vi "Realsense Cam Stream Restart All.vi"(8 "error in (no error)":errorcluster, 11 "Realsense Cam in":refnum<class "Realsense Cam.lvclass">) -> (0 "error out":errorcluster, 3 "Realsense Cam out":refnum<class "Realsense Cam.lvclass">)   [LabVIEW 2018, in "Realsense Cam.lvclass"]
uses:
  Realsense Cam.lvclass
  Realsense Cam.lvclass/Realsense Cam.ctl
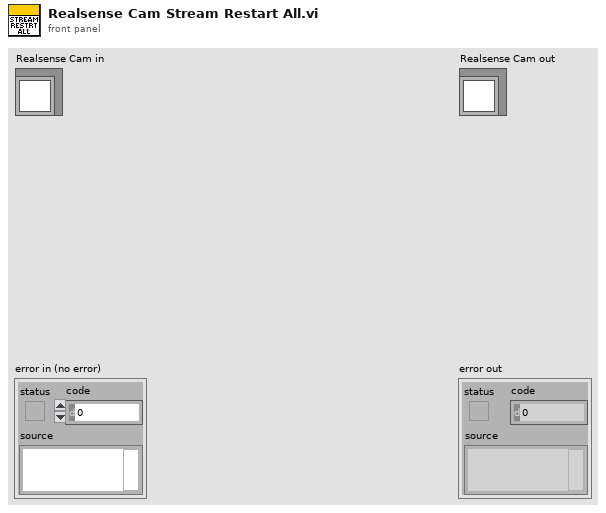
[diagram p1: front panel]
types:
  T1 = cluster{"Depth?":bool, "Left IR?":bool, "Left IR Unrectified?":bool, "Right IR?":bool, "Right IR Unrectified?":bool, "Color?":bool, "RGB Ext.?":bool}
  T2 = typedef "Realsense Cam.lvclass/Activated Stream STYP.ctl" = cluster{"Stream Config":T3, "Profile Handle":u64, "Stream":T5}
  T3 = typedef "Realsense Cam.lvclass/Stream Config STYP.ctl" = cluster{"Stream Type":T4, "Resolution":u16}
  T4 = typedef "Realsense Cam.lvclass/Stream Types Enum STYP.ctl" = enum16{"Depth", "Left IR", "Left IR Unrectified", "Right IR", "Right IR Unrectified", "Color", "RGB Ext."}
  T5 = typedef "Realsense Cam.lvclass/Stream STYP.ctl" = cluster{"Strings":string[], "Intrinsics":cluster{"width":i32, "height":i32, "fps":i32, "Profile":u64, "ppx":sgl, "ppy":sgl, "fx":sgl, "fy":sgl, "model":u32}[], "Current Data":T6}
  T6 = typedef "Realsense Cam.lvclass/Stream Frame Data STYP.ctl" = cluster{"Depths":sgl[][], "Bytes":u8[], "16-Bit IR":u16[], "Height":i32, "Width":i32}
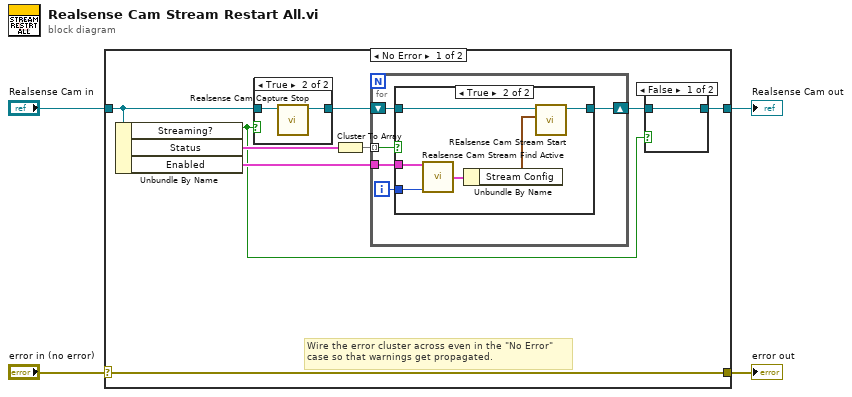
[diagram p0: block diagram]
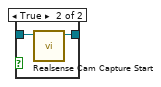
[diagram p2: hidden frame]
diagram:
  n1 = case shown="No Error" "error in (no error)" {
    selector: "error in (no error)" -> [w13 w33]
    tunnel: [w13 w33] -> w3
    tunnel: [w6 w32] -> w1
    tunnel: "Realsense Cam in" -> [w9 w32]
    frame No Error {
      # "Wire the error cluster across even in the \"No Error\"\ncase so that warnings get propagated."
      n2 = Unbundle By Name(w9) -> ("Streaming?"=w5:bool, "Status"=w12:T1, "Enabled"=w10:T2[])
      n3 = case shown="True" w5 {
        tunnel: w9 -> [w17 w19]
        tunnel: [w17 w18] -> w8
        frame False {
        }
        frame True {
          n4 = call-dynamic "Realsense Cam Capture Stop.vi"("Realsense Cam in"=w19) -> ("Realsense Cam out"=w18:refnum<class "Realsense Cam.lvclass">)  [unwired: 8 in, 2 out]
        }
      }
      n5 = Cluster To Array(cluster=w12) -> (array=w11:bool[])
      n6 = for {
        tunnel: w11 -> [w21] mode=indexing
        shift-right: [w20] -> w7
        shift-left: w8 -> [w24]
        tunnel: w10 -> [w23]
        i -> [w22]
        n7 = case shown="True" w21 {
          tunnel: w24 -> [w25 w31]
          tunnel: w23 -> [_ w30]
          tunnel: w22 -> [_ w27]
          tunnel: [w25 w28] -> w20
          frame False {
          }
          frame True {
            n8 = call "Realsense Cam Stream Find Active.vi"("Streams"=w30, "Stream Types"=w27) -> ("Activated Stream"=w29:T2)  [unwired: 11 in, 2 out]
            n9 = Unbundle By Name(w29) -> ("Stream Config"=w26:T3)
            n10 = call-dynamic "REalsense Cam Stream Start.vi"("Stream Config"=w26, "Realsense Cam in"=w31) -> ("Realsense Cam out"=w28:refnum<class "Realsense Cam.lvclass">)  [unwired: 8 in, 1 out]
          }
        }
      }
      n11 = case shown="False" w5 {
        tunnel: w7 -> [w14 w16]
        tunnel: [w14 w15] -> w6
        frame False {
        }
        frame True {
          n12 = call-dynamic "Realsense Cam Capture Start.vi"("Realsense Cam in"=w16) -> ("Realsense Cam out"=w15:refnum<class "Realsense Cam.lvclass">)  [unwired: 8 in, 2 out]
        }
      }
    }
    frame Error {
    }
  }
  "error out" <- w3
  "Realsense Cam out" <- w1
